vi "Compute 1-Exp Guess Parameters.vi"(9 "IRF":cluster{"t Array":dbl[], "Data Array":dbl[]}, 11 "Decay":cluster{"t Array":dbl[], "Data Array":dbl[]}) -> (1 "Ordered Guess Parameter Names":T1[](array[typedef])=[enum."Offset", enum."Baseline", enum."A_1", enum."tau_1"], 3 "Guess Parameters":dbl[](array[numeric]))   [LabVIEW 2021, in "Fits.lvlib"]
uses:
  Fits.lvlib
  IRF(X)PSED/Decay Fit Parameters In List.ctl
  71ad5533-5b84-4c9c-8205-2d3c01e3b80d.vi
  Math/Math.lvlib
  45c1b275-4b46-4fee-884e-ab0f5f209af1.vi
panel:
  # "t0\n\nBL\n\nA\n\ntau"
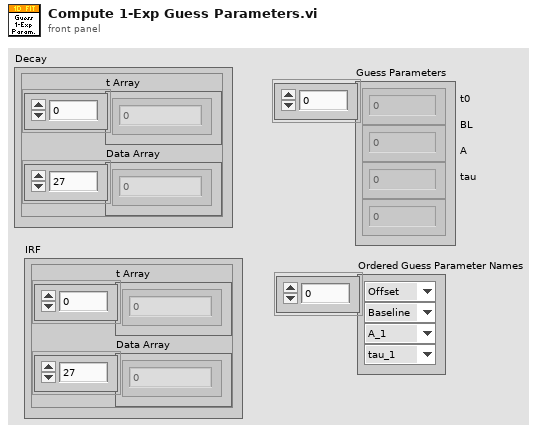
[diagram p1: front panel]
types:
  T1 = typedef "Fits.lvlib/Decay Fit Parameters In List.ctl" = enum16{"Offset", "Baseline", "A_1", "tau_1", "A_2", "tau_2"}
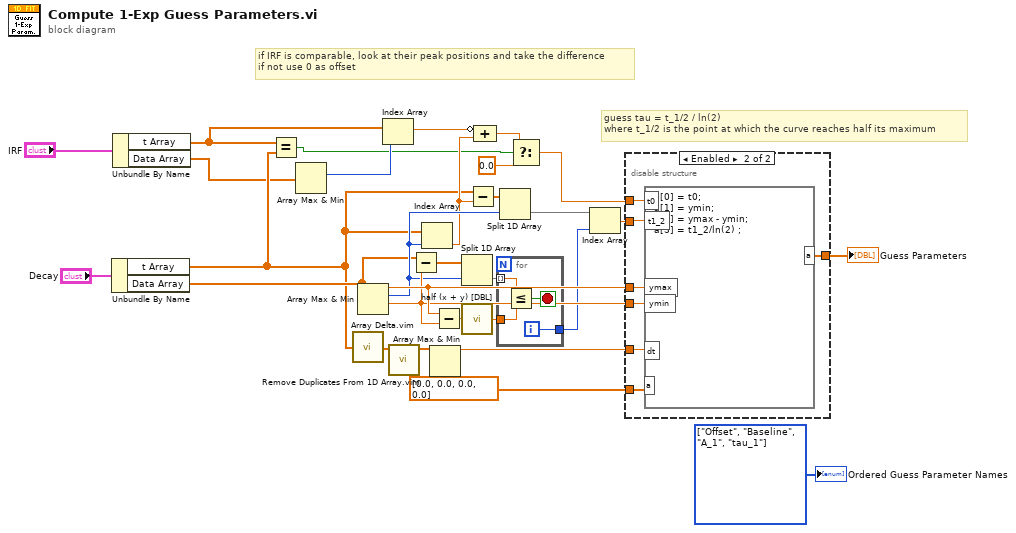
[diagram p0: block diagram]
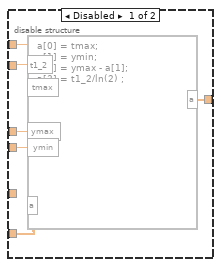
[diagram p2: hidden frame]
diagram:
  w28 = T1[] [enum."Offset", enum."Baseline", enum."A_1", enum."tau_1"] items=["Offset", "Baseline", "A_1", "tau_1", "A_2", "tau_2"] ("data")
  # "if IRF is comparable, look at their peak positions and take the difference\nif not use 0 as offset"
  # "guess tau = t_1/2 / ln(2)\nwhere t_1/2 is the point at which the curve reaches half its maximum"
  n1 = Unbundle By Name("Decay") -> ("t Array"=w5:dbl[], "Data Array"=w13:dbl[])
  n2 = Unbundle By Name("IRF") -> ("t Array"=w11:dbl[], "Data Array"=w3:dbl[])
  n3 = Equal?(x=w11, y=w5) -> (x = y?=w4:bool)
  n4 = Array Max & Min(array=w3) -> (max index (indices)=w10:i32)  [unwired: 3 out]
  n5 = call "Array Delta.vim"("A[i]"=w5) -> ("A[i+1]-A[i]"=w16:dbl[])  [unwired: 8 in]
  n6 = Array Max & Min(array=w13) -> (max value=w26:dbl, max index (indices)=w21:i32, min value=w25:dbl)  [unwired: 1 out]
  n7 = Index Array(array=w11, index=w10) -> (element=w9:dbl)
  n8 = call "Remove Duplicates From 1D Array.vim"("array"=w16) -> ("array with duplicates removed"=w15:dbl[])  [unwired: 10 in]
  n9 = Subtract(x=w13, y=w25) -> (x-y=w27:dbl[])
  n10 = Index Array(array=w5, index=w21) -> (element=w8:dbl)
  n11 = Array Max & Min(array=w15) -> (max value=w14:dbl)  [unwired: 3 out]
  n12 = Subtract(x=w26, y=w25) -> (x-y=w24:dbl)
  n13 = Split 1D Array(array=w27, index=w21) -> (second subarray=w23:dbl[])  [unwired: 1 out]
  n14 = call "half (x + y) [DBL].vi"("x"=w24) -> ("(x+y)/2"=w22:dbl)  [unwired: 5 in]
  n15 = Subtract(x=w5, y=w8) -> (x-y=w19:dbl[])
  n16 = Compound Arithmetic op=ADD(invert w9, w8) -> (w7:dbl)
  n17 = for {
    tunnel: w23 -> [w32] mode=indexing
    tunnel: w22 -> [w34]
    tunnel: [w31] -> w17
    i -> [w31]
    stop <- w33 stop-if-true
    n18 = Less Or Equal?(x=w32, y=w34) -> (x <= y?=w33:bool)
  }
  n19 = Split 1D Array(array=w19, index=w21) -> (second subarray=w20:dbl[])  [unwired: 1 out]
  n20 = Select(t=w7, s=w4, f=0.0) -> (s? t:f=w12:dbl)
  n21 = Index Array(array=w20, index=w17) -> (element=w18:dbl)
  n22 = disable-structure shown="Enabled" {
    disable-tunnel: dbl[] [0.0, 0.0, 0.0, 0.0] ("Guess Parameters") -> [w40 w47]
    disable-tunnel: [w39 w46] -> w29
    disable-tunnel: w26 -> [w38 w45]
    disable-tunnel: w25 -> [w37 w44]
    disable-tunnel: w18 -> [w36 w43]
    disable-tunnel: w12 -> [w35 w42]
    disable-tunnel: w14 -> [_ w41]
    frame Disabled {
      n23 = formula code="a[0] = tmax;\na[1] = ymin;\na[2] = ymax - a[1];\na[3] = t1_2/ln(2) ;"("tmax"=w35, "ymax"=w38, "a"=w40, "ymin"=w37, "t1_2"=w36) -> ("a"=w39:dbl[])
    }
    frame Enabled {
      n24 = formula code="a[0] = t0;\na[1] = ymin;\na[2] = ymax - ymin;\na[3] = t1_2/ln(2) ;"("t0"=w42, "ymax"=w45, "a"=w47, "ymin"=w44, "t1_2"=w43, "dt"=w41) -> ("a"=w46:dbl[])
    }
  }
  "Guess Parameters" <- w29
  "Ordered Guess Parameter Names" <- w28
